vi "LakeShore218_stick_noDB.vi"() -> ()   [LabVIEW 2019]
uses:
  <vilib>/Instr/_visa.llb/VISA Configure Serial Port (Instr).vi
  <vilib>/Utility/file.llb/Write Delimited Spreadsheet (DBL).vi
panel:
  in  "Refresh y scale":bool
  in  "Add 1 hour":bool
  in  "1 hour":bool
  in  "30 minutes":bool
  in  "15 minutes":bool
  in  "5 minutes":bool
  in  "Autoscale time":bool
  in  "Show last (min)":dbl=1.0 min=1.0 step=1.0
  out "r1":dbl format="%_6g"
  out "r2":dbl format="%_6g"
  out "r3":dbl format="%_6g"
  out "r8":dbl format="%_6g"
  out "r7":dbl format="%_6g"
  out "r6":dbl format="%_6g"
  out "r5":dbl format="%_6g"
  out "r4":dbl format="%_6g"
  out "Sensor data":cluster{cluster{"X":dbl, "Y":dbl}[]}[](graph)
  in  "?":bool
  in  "Serial port":refnum<visa-resource-name>
  # "Note: Error codes are assigned negative numbers and status codes are assigned positive numbers."
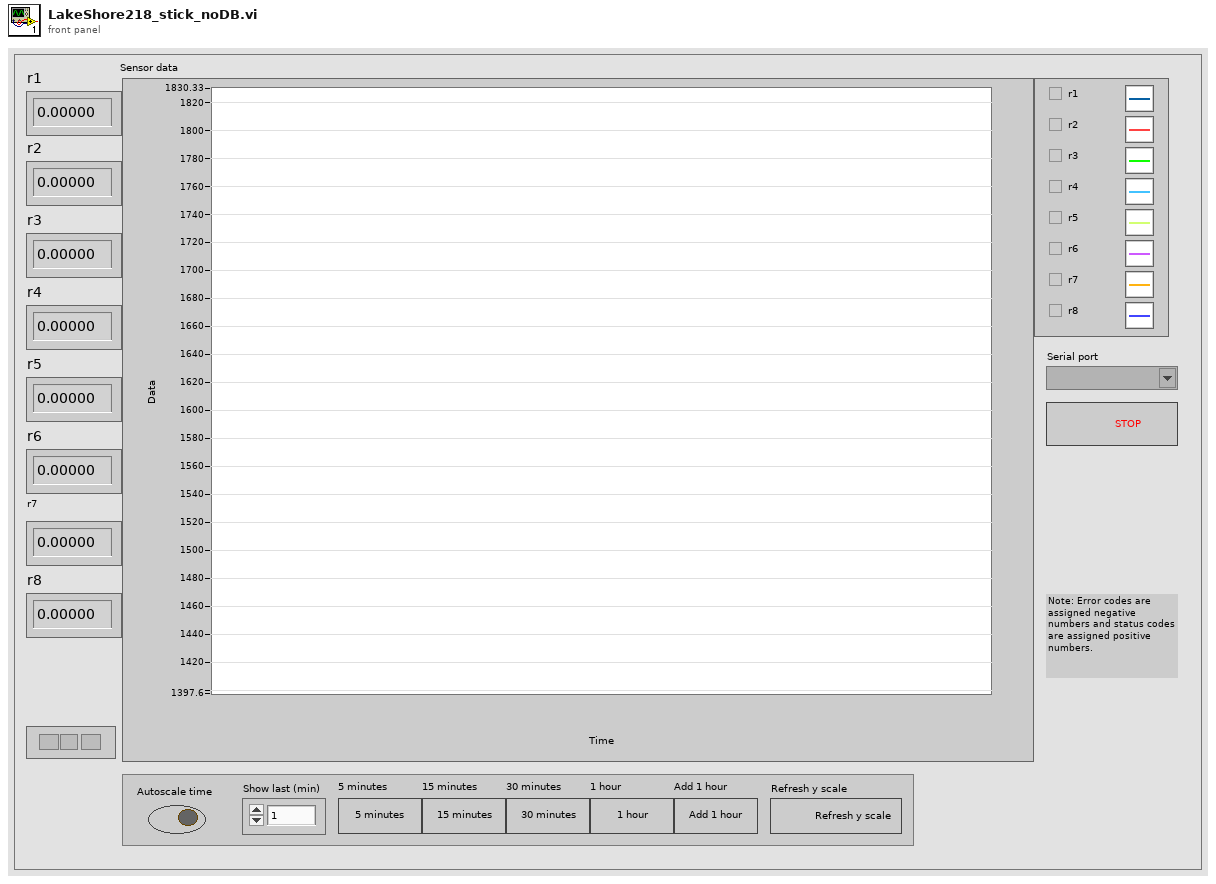
[diagram p1: front panel]
types:
  T1 = typedef "LVRangeTypeDef.ctl" = cluster{"Minimum":dbl, "Maximum":dbl, "Increment":dbl, "Minor Increment":dbl, "Start":dbl}
  T2 = enum8{"Enabled", "Disabled", "Disabled and Grayed Out"}
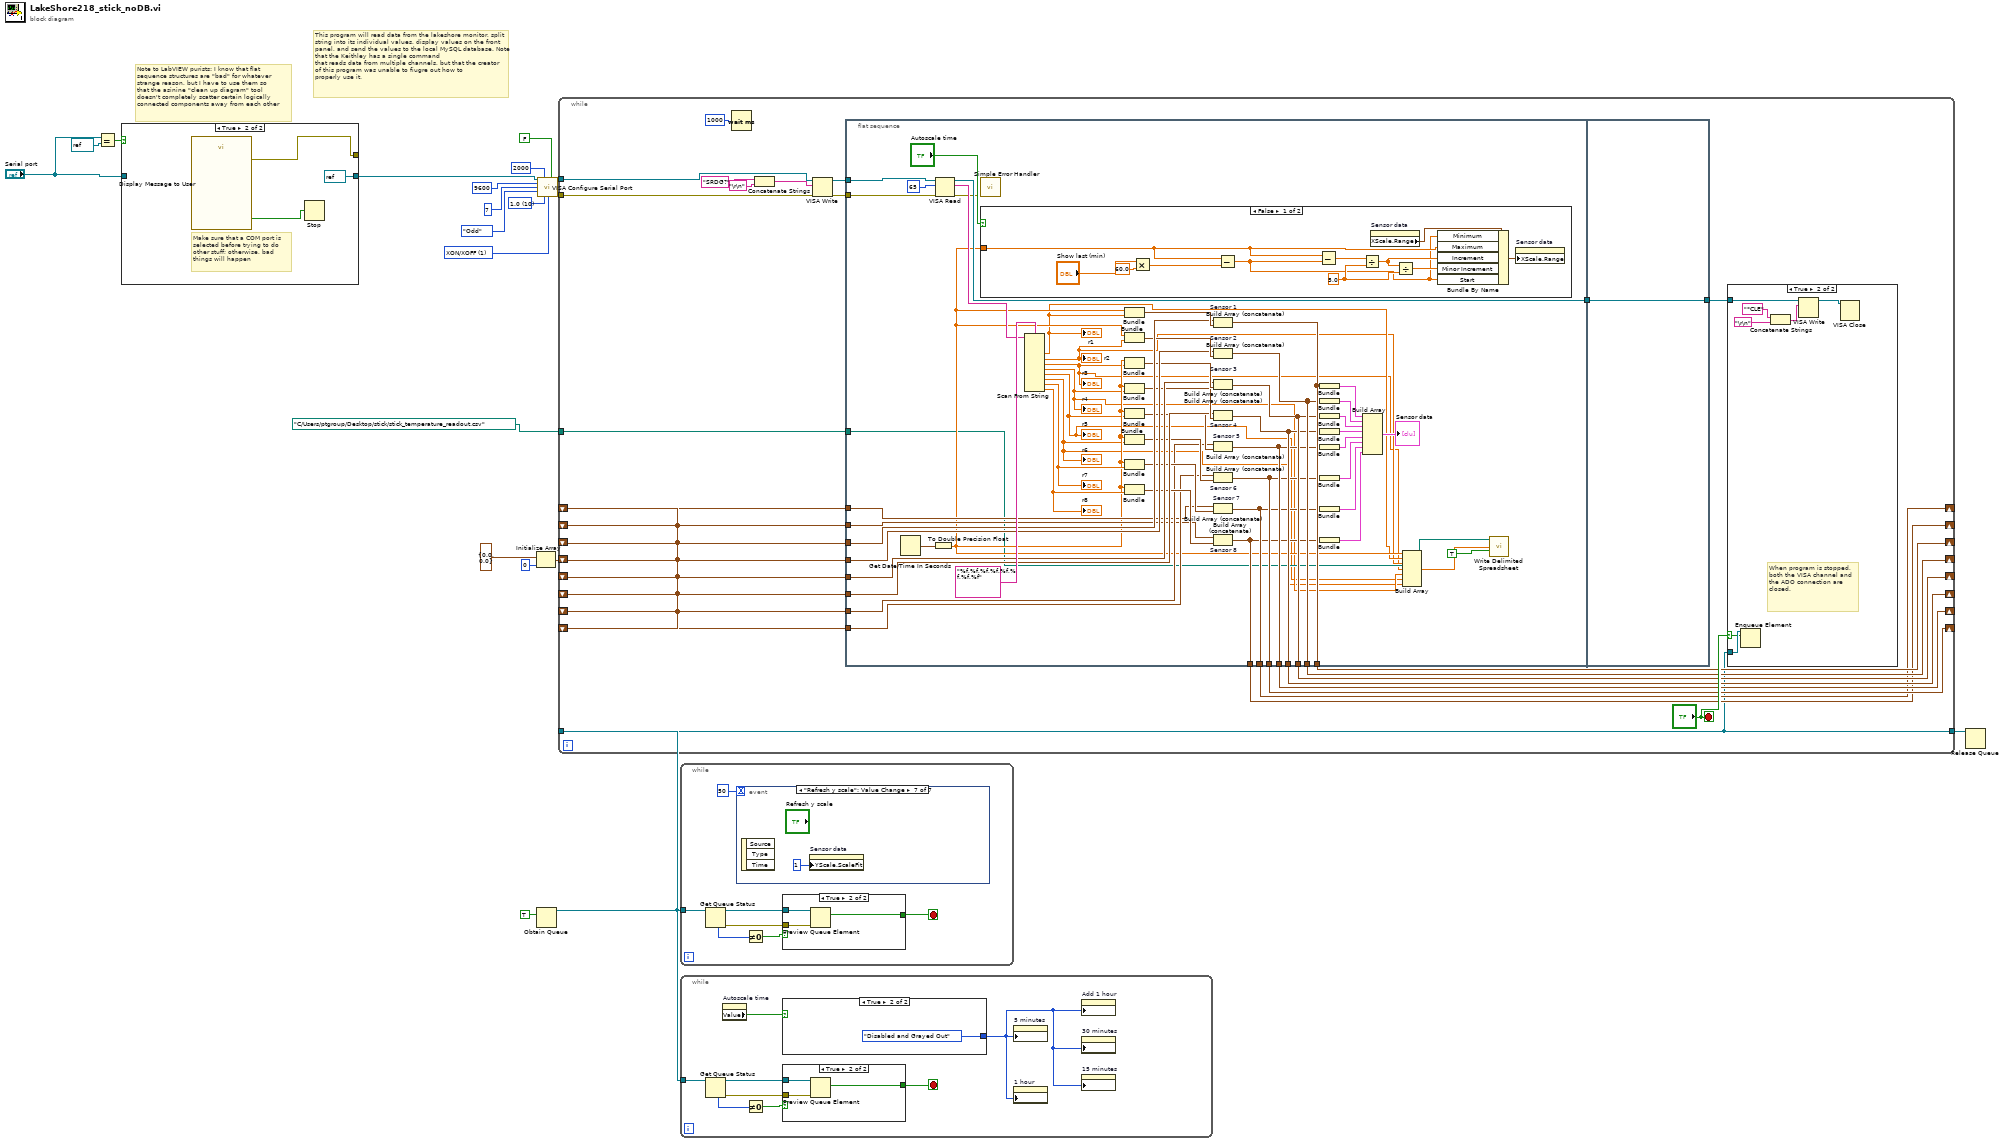
[diagram p0: block diagram]
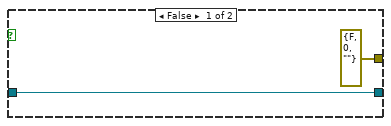
[diagram p2: hidden frame]
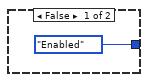
[diagram p3: hidden frame]
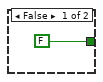
[diagram p4: hidden frame]
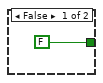
[diagram p5: hidden frame]
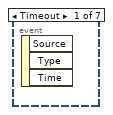
[diagram p6: hidden frame]
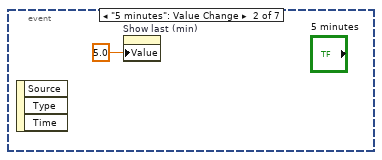
[diagram p7: hidden frame]
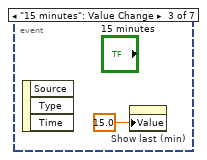
[diagram p8: hidden frame]
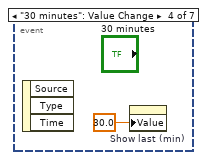
[diagram p9: hidden frame]
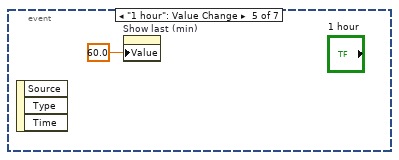
[diagram p10: hidden frame]
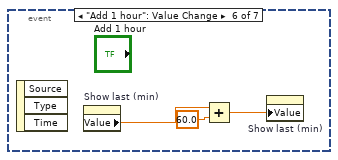
[diagram p11: hidden frame]
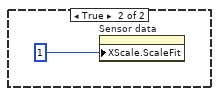
[diagram p13: hidden frame]
diagram:
  w2 = u16 10 items=["1.0"=10, "1.5"=15, "2.0"=20] ("stop bits (10: 1 bit)")
  w13 = u16 1 items=["None", "XON/XOFF", "RTS/CTS", "XON/XOFF & RTS/CTS", "DTR/DSR", "XON/XOFF & DTR/DSR"] ("flow control (0:none)")
  # "Note to LabVIEW purists: I know that flat\nsequence structures are \"bad\" for whatever\nstrange reason, but I have to use them so\nthat the asinine \"clean up diagram\" tool\ndoesn't completely scatter certain logically\nconnected components away from each other"
  # "This program will read data from the lakeshore monitor, split string into its individual values, display values on the front panel, and send the values to the local MySQL database. Note that the Keithley has a single command \nthat reads data from multiple channels, but that the creator of this program was unable to fiugre out how to\nproperly use it."
  n1 = Equal?(x="Serial port", y=refnum<visa-resource-name> refnum) -> (x = y?=w5:bool)
  n2 = case shown="True" w5 {
    tunnel: "Serial port" -> [w22 _]
    tunnel: [w22 refnum<visa-resource-name> refnum ("COM Port")] -> w3
    tunnel: [errorcluster {"status"=FALSE, "code"=0, "source"=""} ("error out") w23] -> _
    frame False {
    }
    frame True {
      # "Make sure that a COM port is\nselected before trying to do\nother stuff; otherwise, bad\nthings will happen"
      n3 = call "Display Message to User"() -> ("error out"=w23:errorcluster, "OK"=w24:bool)  [unwired: 10 in]
      n4 = Stop(stop? (T)=w24) -> ()
    }
  }
  n5 = Initialize Array(cluster{"X":dbl, "Y":dbl} {"X"=0.0, "Y"=0.0}, 0 ("dimension size")) -> (w10:cluster{"X":dbl, "Y":dbl}[])
  n6 = Obtain Queue(element data type=TRUE) -> (queue out=w7:refnum<queue>)  [unwired: 4 in, 2 out]
  n7 = call-poly "VISA Configure Serial Port"("VISA resource name"=w3, "timeout (10sec)"=u32 2000, "Enable Termination\nChar (T)"=FALSE ("Enable Termination\nChar (T)"), "baud rate (9600)"=u32 9600, "data bits (8)"=u16 7, "parity (0:none)"=enum16{"None", "Odd", "Even", "Mark", "Space"}."Odd", "stop bits (10: 1 bit)"=w2, "flow control (0:none)"=w13) -> ("VISA resource name out"=w14:refnum<visa-resource-name>, "error out"=w17:errorcluster)  [unwired: 6 in]
  n8 = while {
    tunnel: w17 -> [w54]
    tunnel: w14 -> [w50]
    shift-right: [w42] -> _
    shift-left: w10 -> [w43]
    shift-right: [w38] -> _
    shift-left: w10 -> [w41]
    shift-right: [w37] -> _
    shift-left: w10 -> [w40]
    shift-right: [w36] -> _
    shift-left: w10 -> [w39]
    shift-right: [w35] -> _
    shift-left: w10 -> [w31]
    shift-right: [w34] -> _
    shift-left: w10 -> [w30]
    shift-right: [w33] -> _
    shift-left: w10 -> [w29]
    shift-right: [w32] -> _
    shift-left: w10 -> [w28]
    tunnel: w7 -> [w27]
    tunnel: [w27] -> w8
    tunnel: path "C:/Users/ptgroup/Desktop/stick/stick_temperature_readout.csv" ("file path (dialog if empty)") -> [w26]
    stop <- "?" stop-if-true
    n9 = Wait (ms)(milliseconds to wait=u32 1000) -> ()  [unwired: 1 out]
    n10 = Concatenate Strings("SRDG?" ("write buffer 2"), "\r\n") -> (w51:string)
    n11 = VISA Write(VISA resource name=w50, write buffer=w51, error in (no error)=w54) -> (VISA resource name out=w49:refnum<visa-resource-name>, error out=w48:errorcluster)  [unwired: 1 out]
    n12 = flat-sequence {
      tunnel: w49 -> [w115]
      tunnel: w48 -> [w114]
      tunnel: [w111] -> w45
      tunnel: w43 -> [w107]
      tunnel: [w106] -> w42
      tunnel: w41 -> [w102]
      tunnel: w40 -> [w99]
      tunnel: w39 -> [w96]
      tunnel: [w84] -> w38
      tunnel: [w83] -> w37
      tunnel: [w82] -> w36
      tunnel: [w81] -> w35
      tunnel: [w80] -> w34
      tunnel: [w79] -> w33
      tunnel: [w78] -> w32
      tunnel: w31 -> [w77]
      tunnel: w30 -> [w76]
      tunnel: w29 -> [w75]
      tunnel: w28 -> [w74]
      tunnel: w26 -> [w66]
      tunnel: [w128] -> w46
      tunnel: w45 -> [w128]
      frame #0 {
        n13 = Get Date/Time In Seconds() -> (seconds since 1Jan1904=w109:timestamp)
        n14 = To Double Precision Float(number=w109) -> (double precision float=w71:dbl)
        n15 = VISA Read(VISA resource name=w115, byte count=u32 65, error in (no error)=w114) -> (VISA resource name out=w111:refnum<visa-resource-name>, read buffer=w110:string, error out=w72:errorcluster)  [unwired: 1 out]
        n16 = call <vilib>:"Simple Error Handler.vi"("error in (no error)"=w72) -> ()  [unwired: 4 in, 5 out]
        n17 = case shown="False" "Autoscale time" {
          tunnel: w71 -> [w123 _]
          frame False {
            w120 = 5.0 ("y")
            n18 = Multiply(x="Show last (min)", y=60.0) -> (x*y=w117:dbl)
            n19 = Subtract(x=w123, y=w117) -> (x-y=w119:dbl)
            n20 = Subtract(x=w123, y=w119) -> (x-y=w124:dbl)
            n21 = Divide(x=w124, y=w120) -> (x/y=w121:dbl)
            n22 = property on="Sensor data" class="XYGraph (strict)"() -> ("XScale.Range"=w126:T1)  [unwired: 2 in, 2 out]
            n23 = Divide(x=w121, y=w120) -> (x/y=w122:dbl)
            n24 = Bundle By Name(cluster=w126, "Minimum"=w119, "Maximum"=w123, "Increment"=w121, "Minor Increment"=w122, "Start"=w119) -> (w125:T1)
            n25 = property on="Sensor data" class="XYGraph (strict)"("XScale.Range"=w125) -> ()  [unwired: 2 in, 2 out]
          }
          frame True {
            n26 = property on="Sensor data" class="XYGraph (strict)"("XScale.ScaleFit"=u8 1 ("X Scale.Scale Fit")) -> ()  [unwired: 2 in, 2 out]
          }
        }
        n27 = Scan From String(format string="%f,%f,%f,%f,%f,%f,%f,%f", input string=w110) -> (output 1=w70:dbl, output 2=w69:dbl, output 3=w65:dbl, output 4=w64:dbl, output 5=w63:dbl, output 6=w62:dbl, output 7=w90:dbl, output 8=w89:dbl)  [unwired: 10 in, 3 out]
        "r4" <- w64
        "r5" <- w63
        "r6" <- w62
        "r7" <- w90
        "r8" <- w89
        "r1" <- w70
        "r2" <- w69
        "r3" <- w65
        n28 = Bundle(w71, "r1"=w70) -> (w108:cluster{dbl, "r1":dbl})  [unwired: 1 in]
        n29 = Bundle(w71, "r2"=w69) -> (w103:cluster{dbl, "r2":dbl})  [unwired: 1 in]
        n30 = Bundle(w71, "r3"=w65) -> (w100:cluster{dbl, "r3":dbl})  [unwired: 1 in]
        n31 = Bundle(w71, "r4"=w64) -> (w97:cluster{dbl, "r4":dbl})  [unwired: 1 in]
        n32 = Bundle(w71, "r5"=w63) -> (w94:cluster{dbl, "r5":dbl})  [unwired: 1 in]
        n33 = Bundle(w71, "r6"=w62) -> (w93:cluster{dbl, "r6":dbl})  [unwired: 1 in]
        n34 = Bundle(w71, "r7"=w90) -> (w92:cluster{dbl, "r7":dbl})  [unwired: 1 in]
        n35 = Bundle(w71, "r8"=w89) -> (w91:cluster{dbl, "r8":dbl})  [unwired: 1 in]
        n36 = Build Array (concatenate) "Sensor 1"(w107, w108) -> (w106:cluster{"X":dbl, "r1":dbl}[])
        n37 = Build Array (concatenate) "Sensor 2"(w102, w103) -> (w84:cluster{"X":dbl, "r2":dbl}[])
        n38 = Build Array (concatenate) "Sensor 3"(w99, w100) -> (w83:cluster{"X":dbl, "r3":dbl}[])
        n39 = Build Array (concatenate) "Sensor 4"(w96, w97) -> (w82:cluster{"X":dbl, "r4":dbl}[])
        n40 = Build Array (concatenate) "Sensor 5"(w77, w94) -> (w81:cluster{"X":dbl, "r5":dbl}[])
        n41 = Build Array (concatenate) "Sensor 6"(w76, w93) -> (w80:cluster{"X":dbl, "r6":dbl}[])
        n42 = Build Array (concatenate) "Sensor 7"(w75, w92) -> (w79:cluster{"X":dbl, "r7":dbl}[])
        n43 = Build Array (concatenate) "Sensor 8"(w74, w91) -> (w78:cluster{"X":dbl, "r8":dbl}[])
        n44 = Bundle(w106) -> (w105:cluster{cluster{"X":dbl, "r1":dbl}[]})  [unwired: 1 in]
        n45 = Bundle(w84) -> (w101:cluster{cluster{"X":dbl, "r2":dbl}[]})  [unwired: 1 in]
        n46 = Bundle(w83) -> (w98:cluster{cluster{"X":dbl, "r3":dbl}[]})  [unwired: 1 in]
        n47 = Bundle(w82) -> (w95:cluster{cluster{"X":dbl, "r4":dbl}[]})  [unwired: 1 in]
        n48 = Bundle(w81) -> (w88:cluster{cluster{"X":dbl, "r5":dbl}[]})  [unwired: 1 in]
        n49 = Bundle(w80) -> (w87:cluster{cluster{"X":dbl, "r6":dbl}[]})  [unwired: 1 in]
        n50 = Bundle(w79) -> (w86:cluster{cluster{"X":dbl, "r7":dbl}[]})  [unwired: 1 in]
        n51 = Bundle(w78) -> (w85:cluster{cluster{"X":dbl, "r8":dbl}[]})  [unwired: 1 in]
        n52 = Build Array(w105, w101, w98, w95, w88, w87, w86, w85) -> (→"Sensor data":cluster{cluster{"X":dbl, "r8":dbl}[]}[])
        n53 = Build Array(w71, w70, w69, w65, w64, w63, w62) -> (w68:dbl[])
        n54 = call-poly <vilib>:"Write Delimited Spreadsheet.vi"("file path (dialog if empty)"=w66, "1D data"=w68, "append to file? (new file:F)"=TRUE ("append to file? (F)")) -> ()  [unwired: 11 in, 2 out]
      }
      frame #1 {
      }
    }
    n55 = case shown="True" "?" {
      selector: "?" -> [_ w56]
      tunnel: w46 -> [_ w58]
      tunnel: w27 -> [_ w57]
      frame False {
      }
      frame True {
        # "When program is stopped,\nboth the VISA channel and\nthe ADO connection are\nclosed."
        n56 = Enqueue Element(queue=w57, element=w56) -> ()  [unwired: 2 in, 3 out]
        n57 = Concatenate Strings("*CLE" ("write buffer 2"), "\r\n") -> (w59:string)
        n58 = VISA Write(VISA resource name=w58, write buffer=w59) -> (VISA resource name out=w55:refnum<visa-resource-name>)  [unwired: 1 in, 2 out]
        n59 = VISA Close(VISA resource name=w55) -> ()  [unwired: 1 in, 1 out]
      }
    }
  }
  n60 = while {
    tunnel: w7 -> [w130]
    stop <- w129 stop-if-true
    n61 = Get Queue Status(queue=w130) -> (queue out=w134:refnum<queue>, error out=w131:errorcluster, # elements in queue=w133:i32)  [unwired: 2 in, 5 out]
    n62 = event shown="[6] \"Refresh y scale\": Value Change" {
      selector: _ -> [_ _ _ _ _ _ _]
      dyn-events: _ -> [_ _ _ _ _ _ _]
      timeout: 50 -> [_ _ _ _ _ _ _]
      event Timeout {
        n63 = event-data() -> ()  [unwired: 1 in, 3 out]
      }
      event "5 minutes": Value Change {
        n64 = event-data() -> ()  [unwired: 1 in, 3 out]
        n65 = property on="Show last (min)" class="DigNum (strict)"("Value"=5.0 ("Show last (min)")) -> ()  [unwired: 2 in, 2 out]
      }
      event "15 minutes": Value Change {
        n66 = event-data() -> ()  [unwired: 1 in, 3 out]
        n67 = property on="Show last (min)" class="DigNum (strict)"("Value"=15.0 ("Show last (min)")) -> ()  [unwired: 2 in, 2 out]
      }
      event "30 minutes": Value Change {
        n68 = event-data() -> ()  [unwired: 1 in, 3 out]
        n69 = property on="Show last (min)" class="DigNum (strict)"("Value"=30.0 ("Show last (min)")) -> ()  [unwired: 2 in, 2 out]
      }
      event "1 hour": Value Change {
        n70 = event-data() -> ()  [unwired: 1 in, 3 out]
        n71 = property on="Show last (min)" class="DigNum (strict)"("Value"=60.0 ("Show last (min)")) -> ()  [unwired: 2 in, 2 out]
      }
      event "Add 1 hour": Value Change {
        n72 = event-data() -> ()  [unwired: 1 in, 3 out]
        n73 = property on="Show last (min)" class="DigNum (strict)"() -> ("Value"=w145:dbl)  [unwired: 2 in, 2 out]
        n74 = Add(x=w145, y=60.0) -> (x+y=w146:dbl)
        n75 = property on="Show last (min)" class="DigNum (strict)"("Value"=w146) -> ()  [unwired: 2 in, 2 out]
      }
      event "Refresh y scale": Value Change {
        n76 = event-data() -> ()  [unwired: 1 in, 3 out]
        n77 = property on="Sensor data" class="XYGraph (strict)"("YScale.ScaleFit"=u8 1 ("Y Scale.Scale Fit")) -> ()  [unwired: 2 in, 2 out]
      }
    }
    n78 = Not Equal To 0?(x=w133) -> (x != 0?=w132:bool)
    n79 = case shown="True" w132 {
      tunnel: w134 -> [_ w139]
      tunnel: [FALSE w138] -> w129
      tunnel: w131 -> [_ w137]
      frame False {
      }
      frame True {
        n80 = Preview Queue Element(queue=w139, error in (no error)=w137) -> (element=w138:bool)  [unwired: 1 in, 3 out]
      }
    }
  }
  n81 = while {
    tunnel: w7 -> [w151]
    stop <- w150 stop-if-true
    n82 = Get Queue Status(queue=w151) -> (queue out=w152:refnum<queue>, error out=w155:errorcluster, # elements in queue=w153:i32)  [unwired: 2 in, 5 out]
    n83 = property on="Autoscale time" class="Bool (strict)"() -> ("Value"=w149:bool)  [unwired: 2 in, 2 out]
    n84 = Not Equal To 0?(x=w153) -> (x != 0?=w154:bool)
    n85 = case shown="True" w149 {
      tunnel: [T2."Enabled" ("Disabled") T2."Disabled and Grayed Out" ("Disabled")] -> w148
      frame False {
      }
      frame True {
      }
    }
    n86 = case shown="True" w154 {
      tunnel: w152 -> [_ w161]
      tunnel: [FALSE w160] -> w150
      tunnel: w155 -> [_ w159]
      frame False {
      }
      frame True {
        n87 = Preview Queue Element(queue=w161, error in (no error)=w159) -> (element=w160:bool)  [unwired: 1 in, 3 out]
      }
    }
    n88 = property on="5 minutes" class="Bool"("DisabledEnum"=w148) -> ()  [unwired: 2 in, 2 out]
    n89 = property on="1 hour" class="Bool"("DisabledEnum"=w148) -> ()  [unwired: 2 in, 2 out]
    n90 = property on="Add 1 hour" class="Bool"("DisabledEnum"=w148) -> ()  [unwired: 2 in, 2 out]
    n91 = property on="30 minutes" class="Bool"("DisabledEnum"=w148) -> ()  [unwired: 2 in, 2 out]
    n92 = property on="15 minutes" class="Bool"("DisabledEnum"=w148) -> ()  [unwired: 2 in, 2 out]
  }
  n93 = Release Queue(queue=w8) -> ()  [unwired: 2 in, 3 out]
